vi "Write Log Messages.vi"(8 "error in (no error)":errorcluster, 10 "Log Messages":string[](array[string]), 11 "Test System in":refnum<class "Test System.lvclass">) -> (0 "error out":errorcluster, 3 "Test System out":refnum<class "Test System.lvclass">)   [LabVIEW 2021, in "Test System.lvclass"]
uses:
  Test System.lvclass
  Test System.lvclass/Test System.ctl
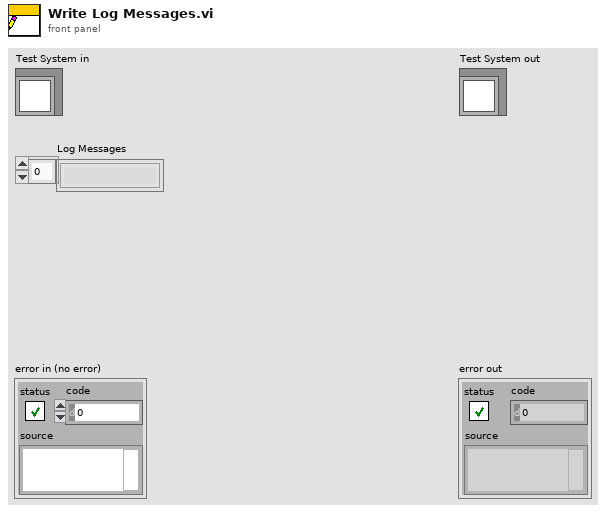
[diagram p1: front panel]
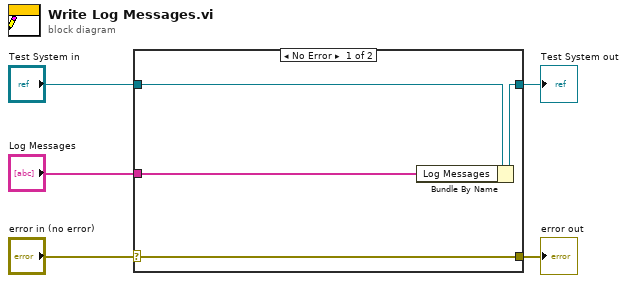
[diagram p0: block diagram]
diagram:
  n1 = case shown="No Error" "error in (no error)" {
    selector: "error in (no error)" -> [w9 w10]
    tunnel: [w9 w10] -> w4
    tunnel: [w7 w11] -> w2
    tunnel: "Test System in" -> [w8 w11]
    tunnel: "Log Messages" -> [w6 _]
    frame No Error {
      n2 = Bundle By Name(cluster=w8, "Log Messages"=w6) -> (w7:refnum<class "Test System.lvclass">)
    }
    frame Error {
    }
  }
  "error out" <- w4
  "Test System out" <- w2
